vi "Auto_Routine_Square.vi"(8 "error in (no error)":errorcluster) -> (0 "error out":errorcluster)   [LabVIEW 2023]
doc: "Drives in a square\n\ninputs:\n--ErrorIn--\noutputs:\n--ErrorOut--"
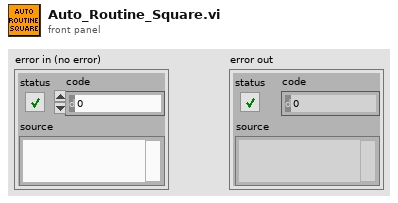
[diagram p1: front panel]
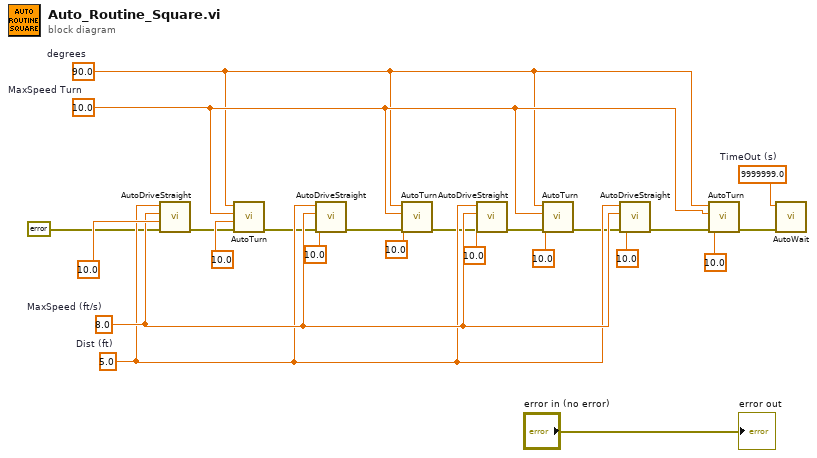
[diagram p0: block diagram]
diagram:
  w15 = 10.0  # MaxSpeed Turn
  w14 = 9999999.0  # TimeOut (s)
  w13 = 90.0  # degrees
  w12 = 8.0  # MaxSpeed (ft/s)
  w11 = 5.0  # Dist (ft)
  n1 = call "AutoDriveStraight.vi"("error in (no error)"=errorcluster {"status"=FALSE, "code"=0, "source"=""}, "TimeOut (s)"=10.0, "MaxSpeed (ft/s)"=w12, "Dist (ft)"=w11) -> ("error out"=w10:errorcluster)  [unwired: 7 in]
  n2 = call "AutoTurn.vi"("error in (no error)"=w10, "TimeOut (s)"=10.0, "MaxSpeed (ft/s)"=w15, "degrees"=w13) -> ("error out"=w9:errorcluster)  [unwired: 7 in]
  n3 = call "AutoDriveStraight.vi"("error in (no error)"=w9, "TimeOut (s)"=10.0, "MaxSpeed (ft/s)"=w12, "Dist (ft)"=w11) -> ("error out"=w8:errorcluster)  [unwired: 7 in]
  n4 = call "AutoTurn.vi"("error in (no error)"=w8, "TimeOut (s)"=10.0, "MaxSpeed (ft/s)"=w15, "degrees"=w13) -> ("error out"=w7:errorcluster)  [unwired: 7 in]
  n5 = call "AutoDriveStraight.vi"("error in (no error)"=w7, "TimeOut (s)"=10.0, "MaxSpeed (ft/s)"=w12, "Dist (ft)"=w11) -> ("error out"=w6:errorcluster)  [unwired: 7 in]
  n6 = call "AutoTurn.vi"("error in (no error)"=w6, "TimeOut (s)"=10.0, "MaxSpeed (ft/s)"=w15, "degrees"=w13) -> ("error out"=w5:errorcluster)  [unwired: 7 in]
  n7 = call "AutoDriveStraight.vi"("error in (no error)"=w5, "TimeOut (s)"=10.0, "MaxSpeed (ft/s)"=w12, "Dist (ft)"=w11) -> ("error out"=w4:errorcluster)  [unwired: 7 in]
  n8 = call "AutoTurn.vi"("error in (no error)"=w4, "TimeOut (s)"=10.0, "MaxSpeed (ft/s)"=w15, "degrees"=w13) -> ("error out"=w3:errorcluster)  [unwired: 7 in]
  n9 = call "AutoWait.vi"("error in (no error)"=w3, "TimeOut (s)"=w14) -> ()  [unwired: 9 in, 1 out]
  "error out" <- "error in (no error)"
